vi "NodeUnderMouse.vi"(8 "error in (no error)":errorcluster, 10 "Coords":T1, 11 "FSM in":refnum<class "FSM.Graph.lvclass">) -> (0 "error out":errorcluster, 1 "contains mouse":bool, 2 "Node":refnum<class "FSM.Node.lvclass">, 3 "Node Index":i32)   [LabVIEW 2015, in "FSM.Graph.lvclass"]
uses:
  FSM.Graph.lvclass
  <vilib>/Utility/miscctls.llb/LVPoint32TypeDef.ctl
  FSM.Node/FSM.Node.lvclass
  FSM.Graph.lvclass/FSM.Graph.ctl
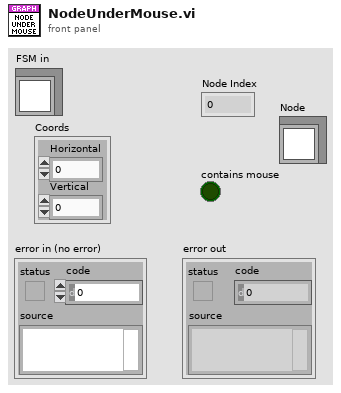
[diagram p1: front panel]
types:
  T1 = typedef "LVPoint32TypeDef.ctl" = cluster{"Horizontal":i32, "Vertical":i32}
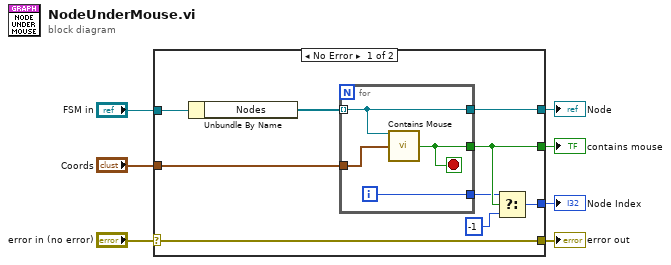
[diagram p0: block diagram]
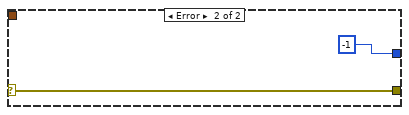
[diagram p2: hidden frame]
diagram:
  n1 = case shown="No Error" "error in (no error)" {
    selector: "error in (no error)" -> [w16 w22]
    tunnel: [w16 w22] -> w6
    tunnel: "FSM in" -> [w15 _]
    tunnel: "Coords" -> [w14 _]
    tunnel: [w11 _] -> w3
    tunnel: [w12 -1] -> w2
    tunnel: [w8 _] -> w1
    frame No Error {
      n2 = Unbundle By Name(w15) -> ("Nodes"=w13:refnum<class "FSM.Node.lvclass">[])
      n3 = for {
        tunnel: w14 -> [w20]
        tunnel: [w19] -> w11
        tunnel: w13 -> [w17] mode=indexing
        tunnel: [w18] -> w10
        tunnel: [w17] -> w8
        i -> [w18]
        stop <- w19 stop-if-true
        n4 = call "Contains Mouse.vi"("FSM.Node"=w17, "Coords"=w20) -> ("contains mouse"=w19:bool)  [unwired: 13 in]
      }
      n5 = Select(t=w10, s=w11, f=-1) -> (s? t:f=w12:i32)
    }
    frame Error {
    }
  }
  "error out" <- w6
  "contains mouse" <- w3
  "Node Index" <- w2
  "Node" <- w1
